vi "Build Minor Frame Instructions.vi"(7 "Virtual Memory Unit in":refnum<class "Virtual Memory Unit.lvclass">, 8 "error in (no error)":errorcluster, 10 "Starting Address":u16 format="%04x", 11 "Minor Frame in":refnum<class "Minor Frame.lvclass">) -> (0 "error out":errorcluster, 2 "Next Available Address":u16 format="%04x", 3 "Minor Frame out":refnum<class "Minor Frame.lvclass">, 5 "Virtual Memory Unit out":refnum<class "Virtual Memory Unit.lvclass">)   [LabVIEW 2020, in "BCI-1553 API.lvlib" / "Minor Frame.lvclass"]
doc: "<DO NOT CALL>\n\nBuilds all the Messages it is responsible for into its subroutine memory block. Afterwards, it will add a mandatory return to make sure execution returns to the Major Frame schedule."
uses:
  Minor Frame.lvclass
  Dependencies/Virtual Memory Unit/Virtual Memory Unit.lvclass
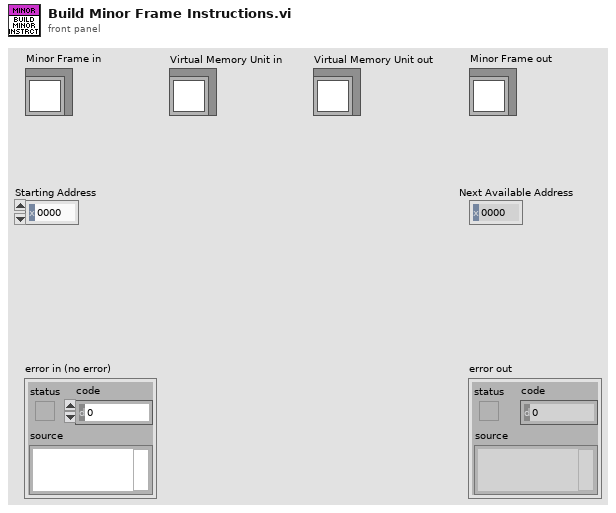
[diagram p1: front panel]
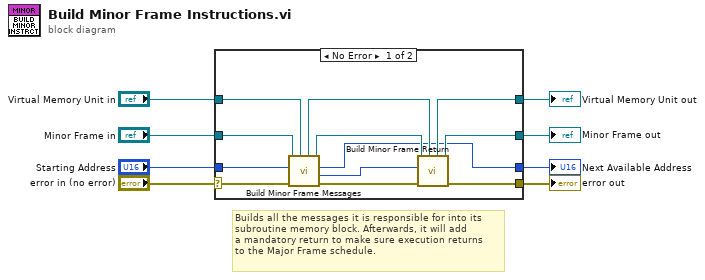
[diagram p0: block diagram]
diagram:
  # "Builds all the messages it is responsible for into its\nsubroutine memory block. Afterwards, it will add\na mandatory return to make sure execution returns\nto the Major Frame schedule."
  n1 = case shown="No Error" "error in (no error)" {
    selector: "error in (no error)" -> [w18 w24]
    tunnel: [w13 w24] -> w7
    tunnel: [w15 w23] -> w5
    tunnel: "Minor Frame in" -> [w19 w23]
    tunnel: [w11 w22] -> w3
    tunnel: "Virtual Memory Unit in" -> [w20 w22]
    tunnel: [w9 w21] -> w2
    tunnel: "Starting Address" -> [w17 w21]
    frame No Error {
      n2 = call "Build Minor Frame Messages.vi"("Virtual Memory Unit in"=w20, "error in (no error)"=w18, "Starting Address"=w17, "Minor Frame in"=w19) -> ("error out"=w14:errorcluster, "Next Available Cmd Address"=w10:u16, "Next Available Data Address"=w9:u16, "Minor Frame out"=w16:refnum<class "Minor Frame.lvclass">, "Virtual Memory Unit out"=w12:refnum<class "Virtual Memory Unit.lvclass">)  [unwired: 3 in]
      n3 = call "Build Minor Frame Return.vi"("Virtual Memory Unit in"=w12, "error in (no error)"=w14, "Starting Address"=w10, "Minor Frame in"=w16) -> ("error out"=w13:errorcluster, "Minor Frame out"=w15:refnum<class "Minor Frame.lvclass">, "Virtual Memory Unit out"=w11:refnum<class "Virtual Memory Unit.lvclass">)  [unwired: 4 in, 1 out]
    }
    frame Error {
    }
  }
  "error out" <- w7
  "Minor Frame out" <- w5
  "Virtual Memory Unit out" <- w3
  "Next Available Address" <- w2
